vi "sub vi - GET ALL TEMP v2.vi"(0 "LA01-EN":bool, 5 "LA02-EN":bool, 7 "LA03-EN":bool, 9 "LA04-EN":bool, 11 "LA05-EN":bool, 12 "Gen Cal Value":dbl) -> (4 "LA01 TEMP":dbl[](array[numeric]), 6 "LA02 TEMP":dbl[](array[numeric]) format="%#.0f", 8 "LA03 TEMP":dbl[](array[numeric]) format="%#.0f", 10 "LA04 TEMP":dbl[](array[numeric]) format="%#.0f", 14 "error":bool, 15 "LA05 TEMP":dbl[](array[numeric]) format="%#.0f")   [LabVIEW 2013]
panel:
  out "LOOP TIME":dbl
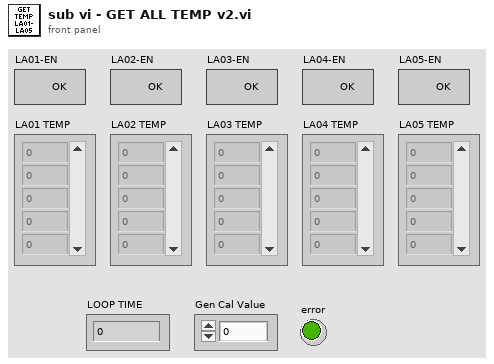
[diagram p1: front panel]
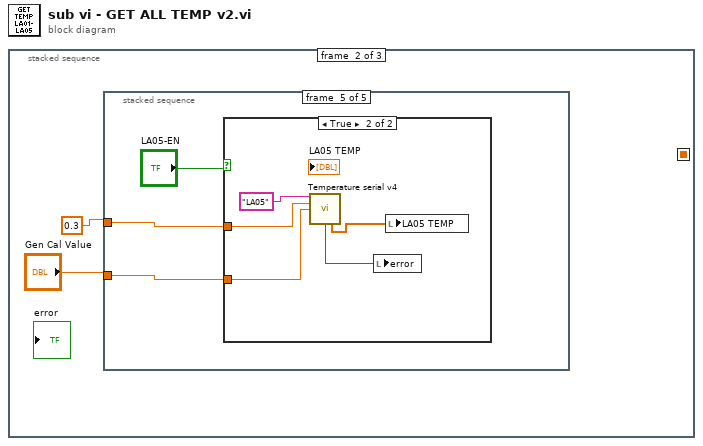
[diagram p0: block diagram]
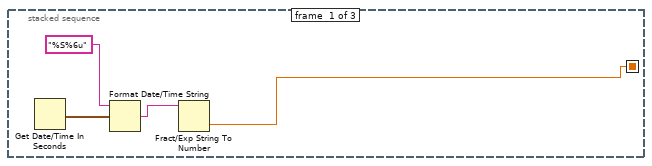
[diagram p2: hidden frame]
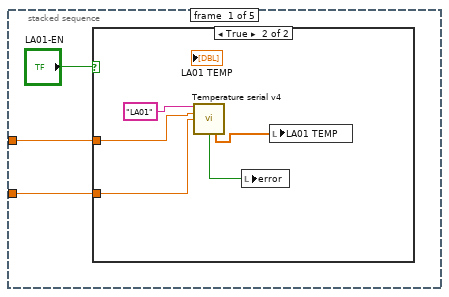
[diagram p3: hidden frame]
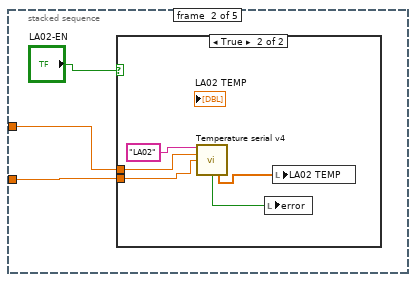
[diagram p5: hidden frame]
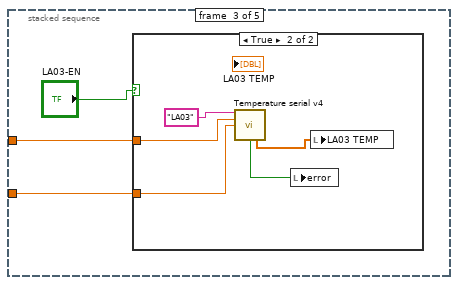
[diagram p7: hidden frame]
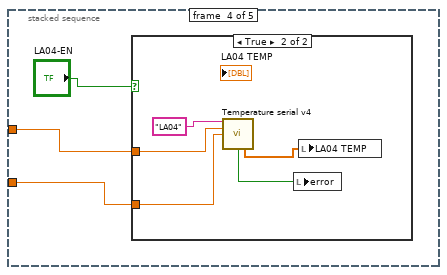
[diagram p9: hidden frame]
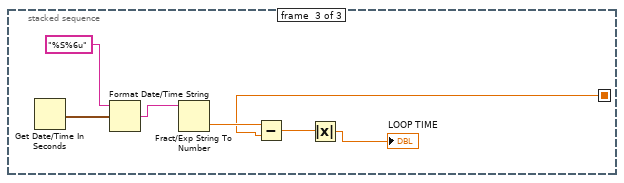
[diagram p12: hidden frame]
diagram:
  n1 = stacked-sequence {
    seq-local: [w1 _ _] -> [_ _ w49]
    frame #0 {
      n2 = Get Date/Time In Seconds() -> (seconds since 1Jan1904=w4:timestamp)
      n3 = Format Date/Time String(time format string (%c)="%S%6u", seconds (now)=w4) -> (date/time string=w2:string)  [unwired: 1 in]
      n4 = Fract/Exp String To Number(string=w2) -> (number=w1:dbl)  [unwired: 3 in, 1 out]
    }
    frame #1 {
      n5 = stacked-sequence {
        tunnel: 0.3 -> [w9 w17 w25 w33 w41]
        tunnel: "Gen Cal Value" -> [w8 w16 w24 w32 w40]
        frame #0 {
          n6 = case shown="True" "LA01-EN" {
            tunnel: w9 -> [_ w13]
            tunnel: w8 -> [_ w11]
            frame False {
            }
            frame True {
              n7 = call "Temperature serial v4.vi"("Command String"="LA01", "Time Out (S)"=w13, "CALIB"=w11) -> ("error"=w10:bool, "Array out"=w12:dbl[])  [unwired: 6 in, 5 out]
              n8 = local write "error"(w10) -> ()
              n9 = local write "LA01 TEMP"(w12) -> ()
            }
          }
        }
        frame #1 {
          n10 = case shown="True" "LA02-EN" {
            tunnel: w17 -> [_ w20]
            tunnel: w16 -> [_ w19]
            frame False {
            }
            frame True {
              n11 = call "Temperature serial v4.vi"("Command String"="LA02", "Time Out (S)"=w20, "CALIB"=w19) -> ("error"=w18:bool, "Array out"=w21:dbl[])  [unwired: 6 in, 5 out]
              n12 = local write "error"(w18) -> ()
              n13 = local write "LA02 TEMP"(w21) -> ()
            }
          }
        }
        frame #2 {
          n14 = case shown="True" "LA03-EN" {
            tunnel: w25 -> [_ w28]
            tunnel: w24 -> [_ w27]
            frame False {
            }
            frame True {
              n15 = call "Temperature serial v4.vi"("Command String"="LA03", "Time Out (S)"=w28, "CALIB"=w27) -> ("error"=w26:bool, "Array out"=w29:dbl[])  [unwired: 6 in, 5 out]
              n16 = local write "error"(w26) -> ()
              n17 = local write "LA03 TEMP"(w29) -> ()
            }
          }
        }
        frame #3 {
          n18 = case shown="True" "LA04-EN" {
            tunnel: w33 -> [_ w36]
            tunnel: w32 -> [_ w35]
            frame False {
            }
            frame True {
              n19 = call "Temperature serial v4.vi"("Command String"="LA04", "Time Out (S)"=w36, "CALIB"=w35) -> ("error"=w34:bool, "Array out"=w37:dbl[])  [unwired: 6 in, 5 out]
              n20 = local write "error"(w34) -> ()
              n21 = local write "LA04 TEMP"(w37) -> ()
            }
          }
        }
        frame #4 {
          n22 = case shown="True" "LA05-EN" {
            tunnel: w41 -> [_ w45]
            tunnel: w40 -> [_ w44]
            frame False {
            }
            frame True {
              n23 = call "Temperature serial v4.vi"("Command String"="LA05", "Time Out (S)"=w45, "CALIB"=w44) -> ("error"=w42:bool, "Array out"=w43:dbl[])  [unwired: 6 in, 5 out]
              n24 = local write "error"(w42) -> ()
              n25 = local write "LA05 TEMP"(w43) -> ()
            }
          }
        }
      }
    }
    frame #2 {
      n26 = Get Date/Time In Seconds() -> (seconds since 1Jan1904=w53:timestamp)
      n27 = Format Date/Time String(time format string (%c)="%S%6u", seconds (now)=w53) -> (date/time string=w51:string)  [unwired: 1 in]
      n28 = Fract/Exp String To Number(string=w51) -> (number=w50:dbl)  [unwired: 3 in, 1 out]
      n29 = Subtract(x=w50, y=w49) -> (x-y=w48:dbl)
      n30 = Absolute Value(x=w48) -> (abs(x)=→"LOOP TIME":dbl)
    }
  }
